vi "CreatePopupWindow.vi"(5 "Offset y":i32, 6 "Flags (SDL_WINDOW_TOOLTIP)":T2=262144 items=["0"=0, "SDL_WINDOW_FULLSCREEN"=1, "SDL_WINDOW_OPENGL"=2, "SDL_WINDOW_OCCLUDED"=4, "SDL_WINDOW_HIDDEN"=8, "SDL_WINDOW_BORDERLESS"=16, "SDL_WINDOW_RESIZABLE"=32, "SDL_WINDOW_MINIMIZED"=64, "SDL_WINDOW_MAXIMIZED"=128, "SDL_WINDOW_MOUSE_GRABBED"=256, "SDL_WINDOW_INPUT_FOCUS"=512, "SDL_WINDOW_MOUSE_FOCUS"=1024, "SDL_WINDOW_EXTERNAL"=2048, "SDL_WINDOW_MODAL"=4096, "SDL_WINDOW_HIGH_PIXEL_DENSITY"=8192, "SDL_WINDOW_MOUSE_CAPTURE"=16384, "SDL_WINDOW_MOUSE_RELATIVE_MODE"=32768, "SDL_WINDOW_ALWAYS_ON_TOP"=65536, "SDL_WINDOW_UTILITY"=131072, "SDL_WINDOW_TOOLTIP"=262144, "SDL_WINDOW_POPUP_MENU"=524288, "SDL_WINDOW_KEYBOARD_GRABBED"=1048576, "SDL_WINDOW_VULKAN"=268435456, "SDL_WINDOW_METAL"=536870912, "SDL_WINDOW_TRANSPARENT"=1073741824, "SDL_WINDOW_NOT_FOCUSABLE"=2147483648], 7 "Offset x":i32, 8 "No Error":errorcluster, 9 "h":i32, 10 "w":i32, 11 "Window [SDL_Window *]":T1 format="%.0x") -> (0 "Error Out":errorcluster, 3 "Popup Window [SDL_Window *]":T1 format="%.0x")   [LabVIEW 2026, in "SDL3.lvlib" / "Video.lvlib"]
doc: "<B>Summary</B>\nCreate a child popup window of the specified parent window.\n\n<B>Remarks</B>\nThe flags parameter must contain at least one of the following:\n- <B>SDL_WINDOW_TOOLTIP</B>: The popup window is a tooltip and will not pass any input events.\n- <B>SDL_WINDOW_POPUP_MENU</B>: The popup window is a popup menu. The topmost popup menu will implicitly gain the keyboard focus.\n\nThe following flags are not relevant to popup window creation and will be ignored:\n<B>SDL_WINDOW_MINIMIZED</B>\n<B>SDL_WINDOW_MAXIMIZED</B>\n<B>SDL_WINDOW_FULLSCREEN</B>\n<B>SDL_WINDOW_BORDERLESS</B>\n\nThe following flags are incompatible with popup window creation and will cause it to fail:\n<B>SDL_WINDOW_UTILITY</B>\n<B>SDL_WINDOW_MODAL</B>\n\nThe parent parameter must be non-null and a valid window. The parent of a popup window can be either a regular, toplevel window, or another popup window.\n\nPopup windows cannot be minimized, maximized, made fullscreen, raised, flash, be made a modal window, be the parent of a toplevel window, or grab the mouse and/or keyboard. Attempts to do so will fail.\n\nPopup windows implicitly do not have a border/decorations and do not appear on the taskbar/dock or in lists of windows such as alt-tab menus.\n\nIf a parent window is hidden or destroyed, any child popup windows will be recursively hidden or destroyed as well. Child popup windows not explicitly hidden will be restored when the parent is shown."
uses:
  Video.lvlib
  WindowFlags--ring.ctl
  <vilib>/Utility/error.llb/Error Cluster From Error Code.vi
  Error/Error.lvlib
  Lib/SDL3.dll
  SDL_Window--pointer.ctl
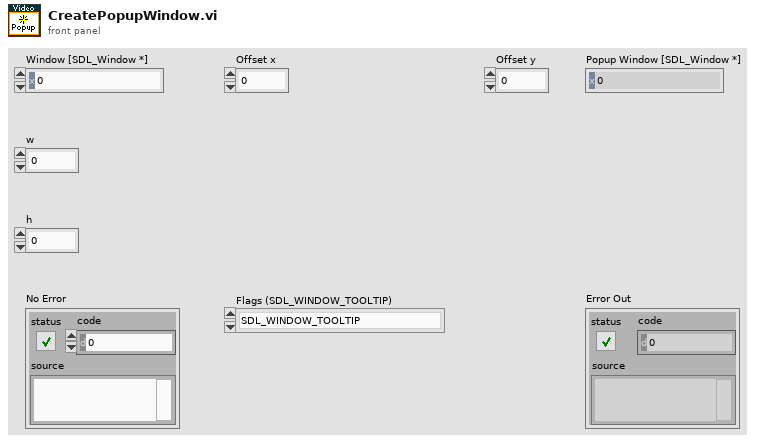
[diagram p1: front panel]
types:
  T1 = typedef "SDL3.lvlib/Video.lvlib/SDL_Window--pointer.ctl" = i64
  T2 = typedef "SDL3.lvlib/Video.lvlib/WindowFlags--ring.ctl" = u64
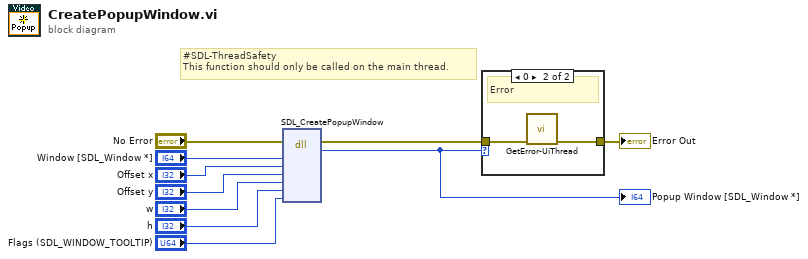
[diagram p0: block diagram]
diagram:
  # "#SDL-ThreadSafety\nThis function should only be called on the main thread."
  n1 = dll-call lib="C:/Users/saukko/Dev/LV-SDL3/Sources/SDL3/Lib/SDL3.*" fn="SDL_CreatePopupWindow"(error in="No Error", "parent"="Window [SDL_Window *]", "offset_x"="Offset x", "offset_y"="Offset y", "w"="w", "h"="h", "flags"="Flags (SDL_WINDOW_TOOLTIP)") -> (error out=w1:errorcluster, "return type"=w6:i64)  [unwired: 8 in, 1 out]
  "Popup Window [SDL_Window *]" <- w6
  n2 = case shown="0" w6 {
    tunnel: w1 -> [w11 w13]
    tunnel: [w11 w12] -> w9
    frame Default {
      # "Ok"
    }
    frame 0 {
      # "Error"
      n3 = call "GetError-UiThread.vi"("No Error"=w13) -> ("error out"=w12:errorcluster)  [unwired: 10 in]
    }
  }
  "Error Out" <- w9
